vi "Kikusui PLZ-Configure Range.vi"(8 "error in":errorcluster, 9 "Range":u16(ring) items=["Low", "Medium", "High"], 10 "Range Type":u16(ring) items=["Current", "Voltage", "Power", "Conductance"], 11 "Kikusui PLZ Setting In":T1={"VISA Resource Name"="", "Baud Rate"=19200, "Stop Bits"=20, "Wait For Read(ms)"=0} {"Stop Bits" items=["1.0"=10, "2.0"=20]; "Baud Rate" items=["2400"=2400, "4800"=4800, "9600"=9600, "19200"=19200]}) -> (0 "error out":errorcluster, 3 "Kikusui PLZ Setting Out":T1={"VISA Resource Name"="", "Baud Rate"=19200, "Stop Bits"=20, "Wait For Read(ms)"=0} {"Stop Bits" items=["1.0"=10, "2.0"=20]; "Baud Rate" items=["2400"=2400, "4800"=4800, "9600"=9600, "19200"=19200]})   [LabVIEW 2018]
doc: "Configures the current, voltage, power or conductance range."
uses:
  Data Def/Kikusui PLZ-Setting.ctl
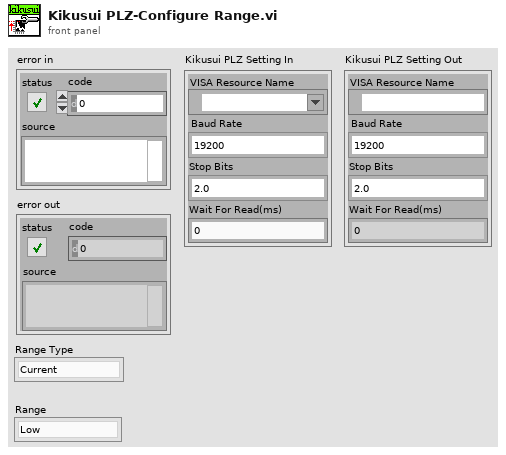
[diagram p1: front panel]
types:
  T1 = typedef "Kikusui PLZ-Setting.ctl" = cluster{"VISA Resource Name":refnum<visa-resource-name>, "Baud Rate":u32, "Stop Bits":u16, "Wait For Read(ms)":u32}
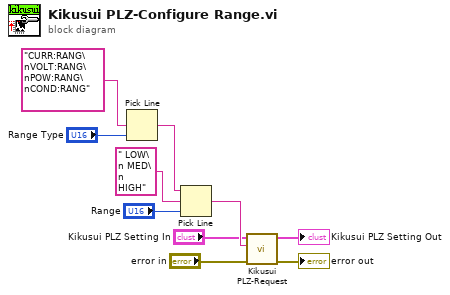
[diagram p0: block diagram]
diagram:
  n1 = Pick Line(multi-line string="CURR:RANG\nVOLT:RANG\nPOW:RANG\nCOND:RANG", line index="Range Type") -> (output string=w9:string)  [unwired: 1 in]
  n2 = Pick Line(string ("")=w9, multi-line string=" LOW\n MED\n HIGH", line index="Range") -> (output string=w4:string)
  n3 = call "Kikusui PLZ-Request.vi"("error in"="error in", "Command"=w4, "Kikusui PLZ Setting In"="Kikusui PLZ Setting In") -> ("error out"=→"error out":errorcluster, "Kikusui PLZ Setting Out"=→"Kikusui PLZ Setting Out":T1)  [unwired: 6 in, 1 out]
